vi "Tear Down TS.vi"(8 "error in":errorcluster, 11 "DeepU Test Stand in":refnum<class "DeepU Test Stand.lvclass">) -> (0 "error out":errorcluster, 3 "DeepU Test Stand out":refnum<class "DeepU Test Stand.lvclass">)   [LabVIEW 2019, in "Test Stands.lvlib" / "DeepU Test Stand.lvclass"]
uses:
  DeepU Test Stand.lvclass
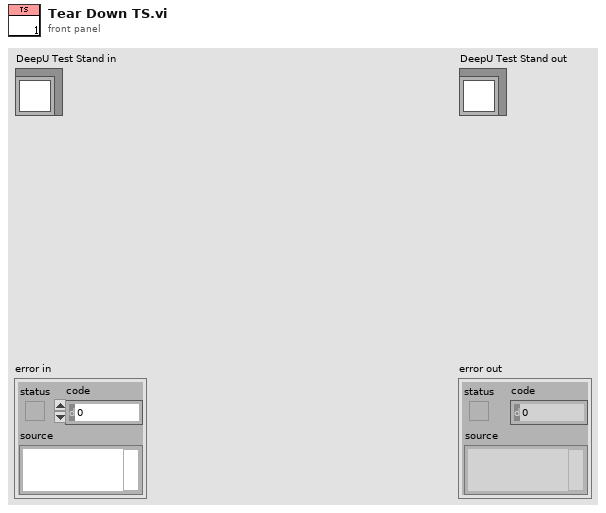
[diagram p1: front panel]
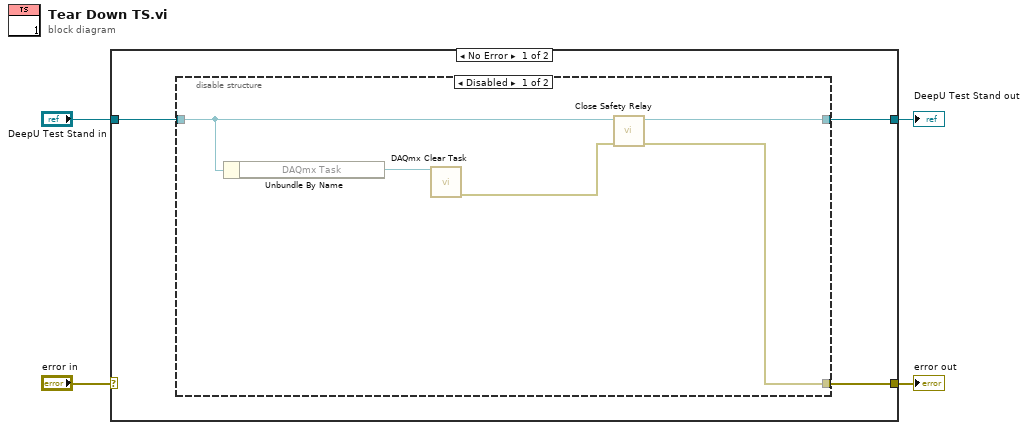
[diagram p0: block diagram]
diagram:
  n1 = case shown="No Error" "error in" {
    selector: "error in" -> [_ w15]
    tunnel: [w6 w15] -> w4
    tunnel: [w7 w14] -> w3
    tunnel: "DeepU Test Stand in" -> [w5 w14]
    frame No Error {
      n2 = disable-structure shown="Disabled" {
        disable-tunnel: [w12 w13] -> w7
        disable-tunnel: [w11 _] -> w6
        disable-tunnel: w5 -> [w10 w13]
        frame Disabled {
          n3 = Unbundle By Name(w10) -> ("DAQmx Task"=w9:refnum<k21>)
          n4 = call <vilib>:"DAQmx Clear Task.vi"("task in"=w9) -> ("error out"=w8:errorcluster)  [unwired: 14 in]
          n5 = call "Close Safety Relay.vi"("error in (no error)"=w8, "DeepU Test Stand in"=w10) -> ("error out"=w11:errorcluster, "DeepU Test Stand out"=w12:refnum<class "DeepU Test Stand.lvclass">)  [unwired: 8 in]
        }
        frame Enabled {
        }
      }
    }
    frame Error {
    }
  }
  "error out" <- w4
  "DeepU Test Stand out" <- w3
